vi "Write.vi"(8 "error in (no error)":errorcluster, 9 "Variant":variant, 10 "String":string, 11 "RS232 in":refnum<class "RS-xxx.lvclass">) -> (0 "error out":errorcluster, 3 "RS232 out":refnum<class "RS-xxx.lvclass">)   [LabVIEW 2013, in "Protocol Classes.lvlib" / "RS-xxx.lvclass"]
uses:
  RS-xxx.lvclass
  RS-xxx.lvclass/RS-xxx.ctl
  Data Access/Read Port Ref.vi
  Data Access/Write Port Ref.vi
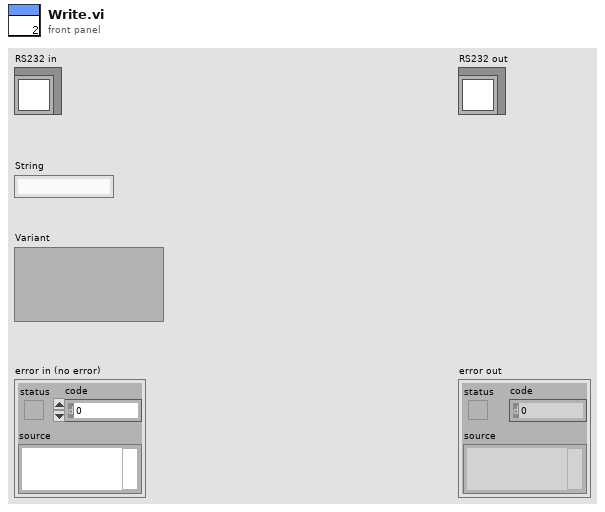
[diagram p1: front panel]
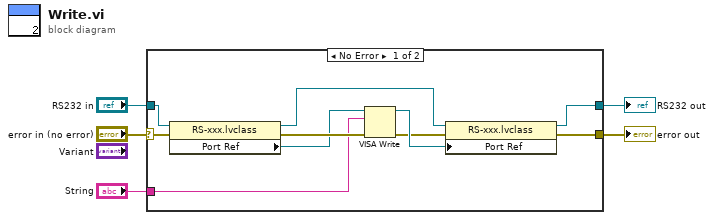
[diagram p0: block diagram]
diagram:
  n1 = case shown="No Error" "error in (no error)" {
    selector: "error in (no error)" -> [w6 w17]
    tunnel: "RS232 in" -> [w15 w16]
    tunnel: "String" -> [w13 _]
    tunnel: [w9 w17] -> w3
    tunnel: [w7 w16] -> w2
    frame No Error {
      n2 = property class="RS-xxx.lvclass"(reference=w15, error in=w6) -> (reference out=w8:refnum<class "RS-xxx.lvclass">, error out=w14:errorcluster, "Port Ref"=w12:refnum<visa-resource-name>)
      n3 = VISA Write(VISA resource name=w12, write buffer=w13, error in (no error)=w14) -> (VISA resource name out=w11:refnum<visa-resource-name>, error out=w10:errorcluster)  [unwired: 1 out]
      n4 = property class="RS-xxx.lvclass"(reference=w8, error in=w10, "Port Ref"=w11) -> (reference out=w7:refnum<class "RS-xxx.lvclass">, error out=w9:errorcluster)
    }
    frame Error {
    }
  }
  "error out" <- w3
  "RS232 out" <- w2
